vi "Pad x410 data.vi"(11 "Data":dbl[][](array[numeric])) -> (3 "Padded data":dbl[][](array[numeric]))   [LabVIEW 2025]
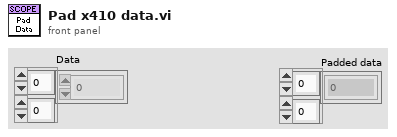
[diagram p1: front panel]
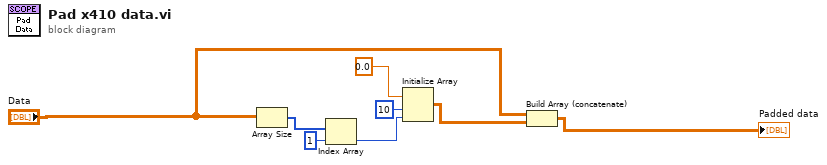
[diagram p0: block diagram]
diagram:
  n1 = Array Size(array="Data") -> (size(s)=w8:i32[])
  n2 = Index Array(array=w8, index=1) -> (element=w5:i32)
  n3 = Initialize Array(0.0 ("element"), 10 ("dimension size"), w5) -> (w3:dbl[][])
  n4 = Build Array (concatenate)("Data", w3) -> (→"Padded data":dbl[][])
